vi "remove current subpanel.vi"(8 "error in":errorcluster, 9 "current VI":refnum<vi>, 10 "stop":refnum<user-event>, 11 "SubPanel in":refnum<vi>) -> (0 "error out":errorcluster)   [LabVIEW 2013, in "vi mod UI.lvlib"]
uses:
  vi mod UI.lvlib
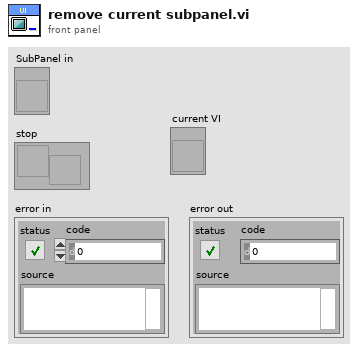
[diagram p1: front panel]
types:
  T1 = enum32{"Bad", "Idle", "Run top level", "Running"}
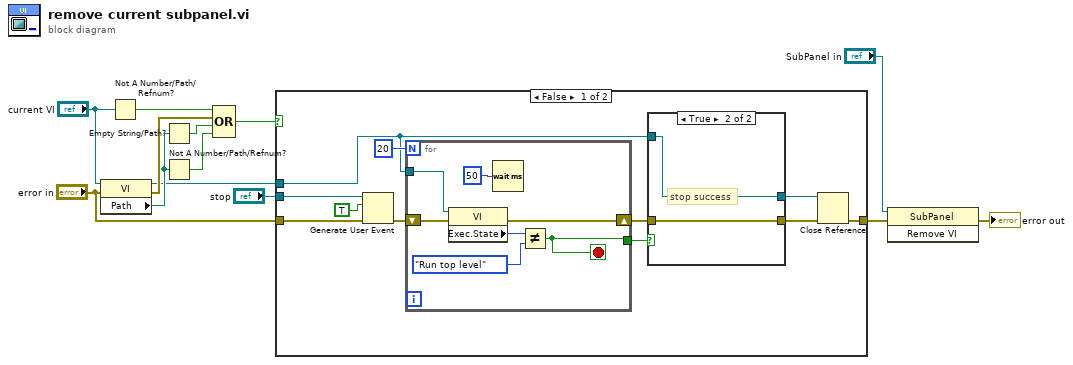
[diagram p0: block diagram]
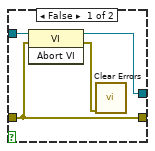
[diagram p2: hidden frame]
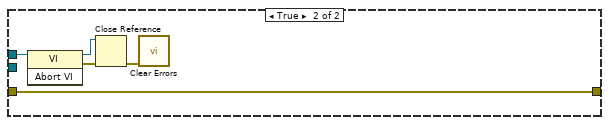
[diagram p3: hidden frame]
diagram:
  n1 = property class="VI"(reference="current VI", error in="error in") -> (reference out=w5:refnum<vi>, error out=w13:errorcluster, "Path"=w10:path)
  n2 = Not A Number/Path/Refnum?(number/path/refnum="current VI") -> (NaN/Path/Refnum?=w9:bool)
  n3 = Empty String/Path?(string/path=w10) -> (empty?=w12:bool)
  n4 = Not A Number/Path/Refnum?(number/path/refnum=w10) -> (NaN/Path/Refnum?=w11:bool)
  n5 = Compound Arithmetic op=OR(w9, w13, w12, w11) -> (w8:bool)
  n6 = case shown="False" w8 {
    tunnel: "error in" -> [w24 w42]
    tunnel: "stop" -> [w23 _]
    tunnel: w5 -> [w16 w41]
    tunnel: [w15 w42] -> w4
    frame False {
      n7 = Generate User Event(user event=w23, event data cluster=TRUE ("event data"), error in=w24) -> (error out=w20:errorcluster)  [unwired: 1 in, 1 out]
      n8 = for {
        N: 20 -> [_]
        tunnel: w16 -> [w37]
        tunnel: [w33] -> w19
        shift-right: [w31] -> w17
        shift-left: w20 -> [w32]
        stop <- w33 stop-if-true
        n9 = property class="VI"(reference=w37, error in=w32) -> (error out=w31:errorcluster, "Exec.State"=w34:T1)  [unwired: 1 out]
        n10 = Wait (ms)(milliseconds to wait=u32 50) -> ()  [unwired: 1 out]
        n11 = Not Equal?(x=w34, y=T1."Run top level") -> (x != y?=w33:bool)
      }
      n12 = case shown="True" w19 {
        tunnel: [w26 w30] -> w18
        tunnel: w17 -> [w26 w30]
        tunnel: w16 -> [w28 w29]
        tunnel: [w25 w29] -> w14
        frame False {
          n13 = invoke class="VI" method="Abort VI"(reference=w28, error in=w26) -> (reference out=w25:refnum<vi>, error out=w27:errorcluster)  [unwired: 1 in, 1 out]
          n14 = call <vilib>:"Clear Errors.vi"("error in (no error)"=w27) -> ()  [unwired: 6 in, 1 out]
        }
        frame True {
          # "stop success"
        }
      }
      n15 = Close Reference(reference=w14, error in (no error)=w18) -> (error out=w15:errorcluster)
    }
    frame True {
      n16 = invoke class="VI" method="Abort VI"(reference=w41) -> (reference out=w38:refnum<vi>, error out=w40:errorcluster)  [unwired: 2 in, 1 out]
      n17 = Close Reference(reference=w38, error in (no error)=w40) -> (error out=w39:errorcluster)
      n18 = call <vilib>:"Clear Errors.vi"("error in (no error)"=w39) -> ()  [unwired: 6 in, 1 out]
    }
  }
  n19 = invoke on="Invoke Node" class="SubPanel" method="Remove VI"(reference="SubPanel in", error in=w4) -> (error out=→"error out":errorcluster)  [unwired: 1 in, 2 out]
